vi "get single issue via cv_api.vi"() -> ()   [LabVIEW 2024]
uses:
  CV_RESTful_Library/CV_RESTful_Lib.lvlib
  <vilib>/addons/_JKI.lib/REST Client/classes/REST Client/REST Client.lvclass
  CV_RESTful_Library/typedefs/cv_issue.generic_credit--cluster.ctl
  CV_RESTful_Library/typedefs/cv_issue.person_credit--cluster.ctl
  CV_RESTful_Library/typedefs/cv_issue.associated_image--cluster.ctl
  CV_RESTful_Library/typedefs/local_issue--cluster.ctl
panel:
  in  "issue id":i32
  out "local_issue":T1
  out "error out":errorcluster
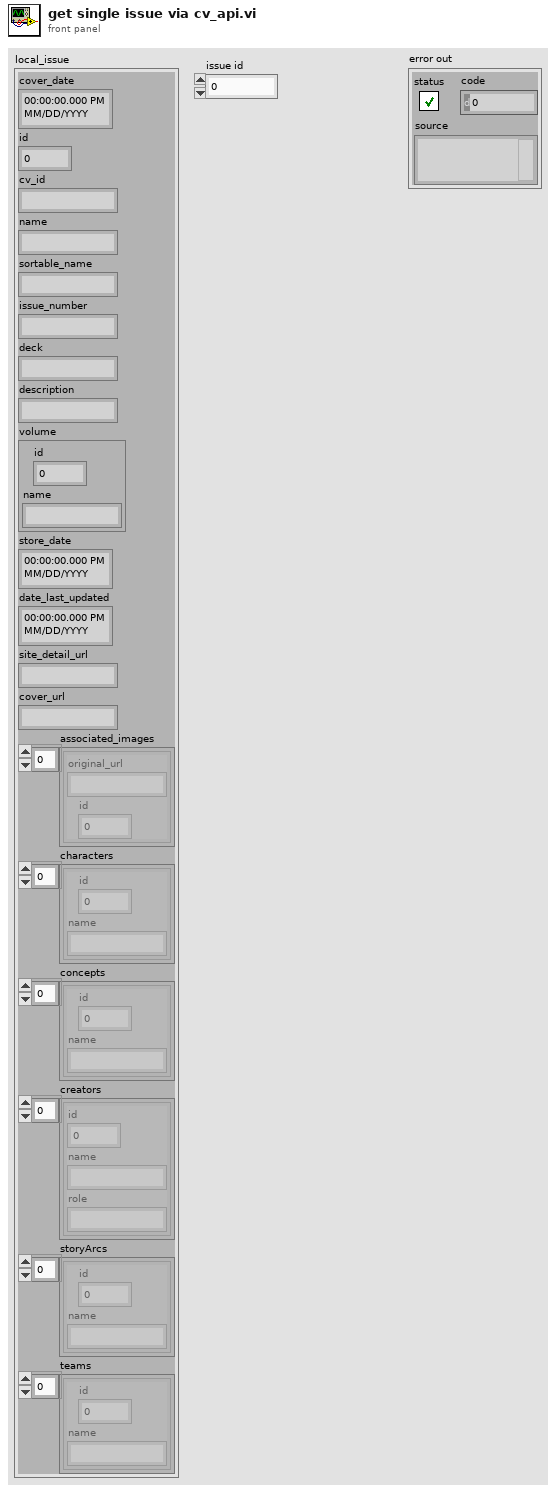
[diagram p1: front panel]
types:
  T1 = typedef "CV_RESTful_Lib.lvlib/local_issue--cluster.ctl" = cluster{"cover_date":timestamp, "id":i32, "cv_id":string, "name":string, "sortable_name":string, "issue_number":string, "deck":string, "description":string, "volume":T2, "store_date":timestamp, "date_last_updated":timestamp, "site_detail_url":string, "cover_url":string, "associated_images":T3[], "characters":T2[], "concepts":T2[], "creators":T4[], "storyArcs":T2[], "teams":T2[]}
  T2 = typedef "CV_RESTful_Lib.lvlib/cv_issue.generic_credit--cluster.ctl" = cluster{"id":i32, "name":string}
  T3 = typedef "CV_RESTful_Lib.lvlib/cv_issue.associated_image--cluster.ctl" = cluster{"original_url":string, "id":i32}
  T4 = typedef "CV_RESTful_Lib.lvlib/cv_issue.person_credit--cluster.ctl" = cluster{"id":i32, "name":string, "role":string}
  T5 = typedef "CV_RESTful_Lib.lvlib/local_issue.ctl" = cluster{"cover_date":timestamp, "id":i32, "cv_id":string, "name":string, "sortable_name":string, "issue_number":string, "deck":string, "description":string, "volume":T2, "store_date":timestamp, "date_last_updated":timestamp, "site_detail_url":string, "cover_url":string, "associated_images":T3[], "characters":T2[], "concepts":T2[], "creators":T4[], "storyArcs":T2[], "teams":T2[]}
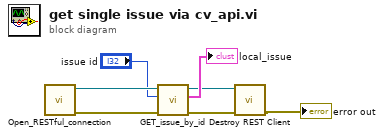
[diagram p0: block diagram]
diagram:
  n1 = call "Open_RESTful_connection.vi"() -> ("error out"=w6:errorcluster, "REST Client out"=w7:refnum<class "REST Client.lvclass">)  [unwired: 10 in]
  n2 = call "GET_issue_by_id.vi"("error in (no error)"=w6, "issue id"="issue id", "REST Client in"=w7) -> ("error out"=w2:errorcluster, "local_issue"=→"local_issue":T5, "REST Client out"=w3:refnum<class "REST Client.lvclass">)  [unwired: 6 in]
  n3 = call-dynamic "Destroy REST Client.vi"("error in (no error)"=w2, "REST Client in"=w3) -> ("error out"=→"error out":errorcluster)  [unwired: 9 in]
